vi "anothermodule.vi"(9 "Numeric":i32, 10 "Numeric 2":i32, 11 "Array":refnum<vi>[][](array[refnum])) -> (3 "Boolean":bool)   [LabVIEW 2014]
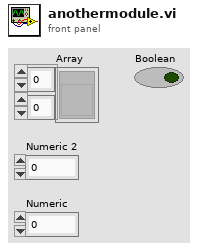
[diagram p1: front panel]
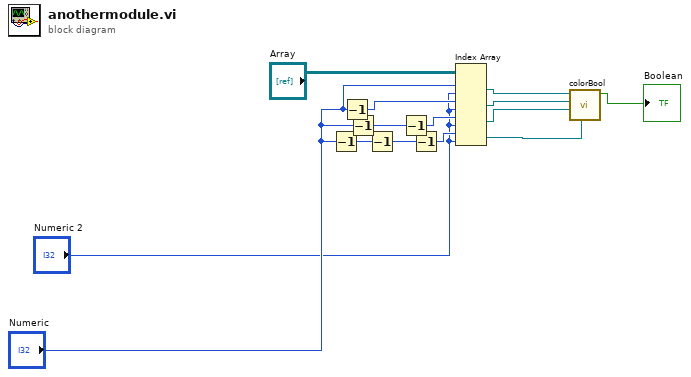
[diagram p0: block diagram]
diagram:
  n1 = Decrement(x="Numeric") -> (x-1=w8:i32)
  n2 = Decrement(x="Numeric") -> (x-1=w3:i32)
  n3 = Decrement(x="Numeric") -> (x-1=w7:i32)
  n4 = Decrement(x=w8) -> (x-1=w9:i32)
  n5 = Decrement(x=w7) -> (x-1=w4:i32)
  n6 = Decrement(x=w9) -> (x-1=w5:i32)
  n7 = Index Array(array="Array", index (row) #1="Numeric", index (col) #1="Numeric 2", index (row) #2=w3, index (col) #2="Numeric 2", index (row) #3=w4, index (col) #3="Numeric 2", index (row) #4=w5, index (col) #4="Numeric 2") -> (element #1=w10:refnum<vi>, element #2=w11:refnum<vi>, element #3=w12:refnum<vi>, element #4=w13:refnum<vi>)
  n8 = call "colorBool.vi"("GObj Refnum"=w13, "GObj Refnum 2"=w12, "GObj Refnum 3"=w11, "GObject in"=w10) -> ("Boolean"=→"Boolean":bool)  [unwired: 7 in]
